vi "XY.vi"() -> ()   [LabVIEW 2017]
panel:
  out "XY Graph":cluster{dbl[], dbl[]}(graph)
  in  "Knob":dbl(knob) scale=0.0..600.0
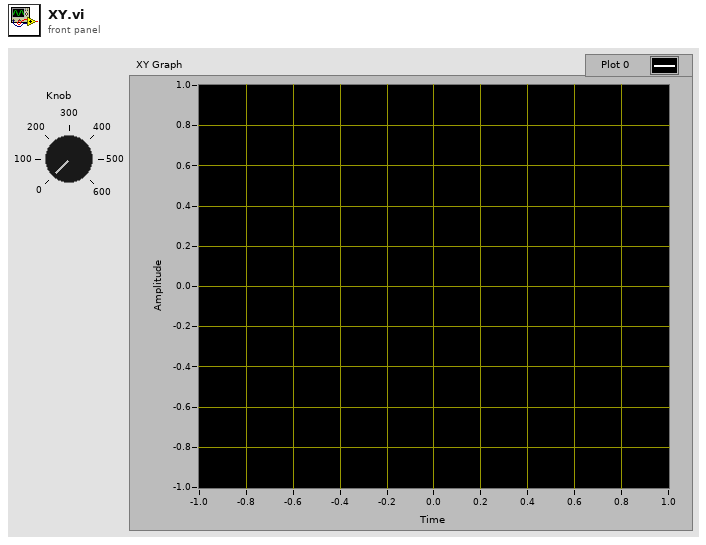
[diagram p1: front panel]
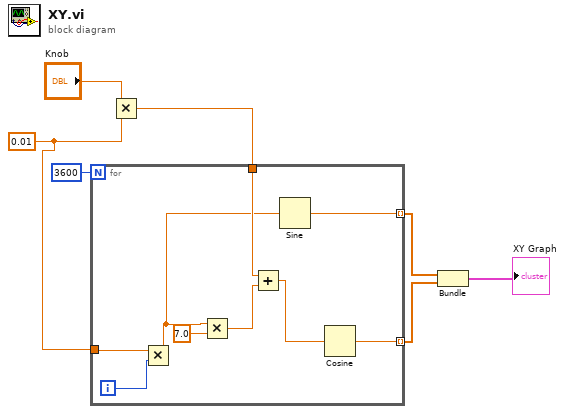
[diagram p0: block diagram]
diagram:
  w5 = 0.01
  n1 = Multiply(x="Knob", y=w5) -> (x*y=w4:dbl)
  n2 = for {
    N: 3600 -> [_]
    tunnel: w5 -> [w15]
    tunnel: w4 -> [w14]
    tunnel: [w9] -> w1 mode=indexing
    tunnel: [w8] -> w2 mode=indexing
    i -> [w16]
    n3 = Multiply(x=w15, y=w16) -> (x*y=w11:dbl)
    n4 = Multiply(x=w11, y=7.0) -> (x*y=w12:dbl)
    n5 = Add(x=w14, y=w12) -> (x+y=w10:dbl)
    n6 = Sine(x=w11) -> (sin(x)=w9:dbl)
    n7 = Cosine(x=w10) -> (cos(x)=w8:dbl)
  }
  n8 = Bundle(w1, w2) -> (→"XY Graph":cluster{dbl[], dbl[]})  [unwired: 1 in]
